vi "GetPort.vi"(8 "error in (no error)":errorcluster, 10 "Port":u8, 11 "NXP LPCXpresso54608 in":refnum<class "NXP LPCXpresso54608.lvclass">) -> (0 "error out":errorcluster, 1 "Response":string, 2 "Value":u8, 3 "NXP LPCXpresso54608 out":refnum<class "NXP LPCXpresso54608.lvclass">)   [LabVIEW 2020, in "NXP LPCXpresso54608.lvclass"]
doc: "Get the status of a digital port on the target device."
uses:
  NXP LPCXpresso54608.lvclass
  MCU/MCU.lvclass
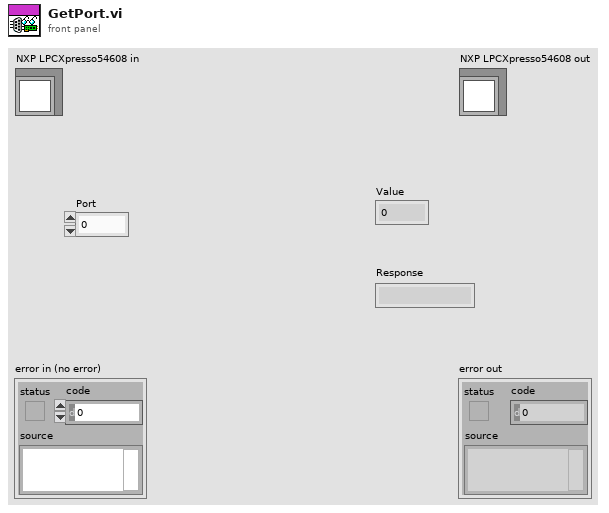
[diagram p1: front panel]
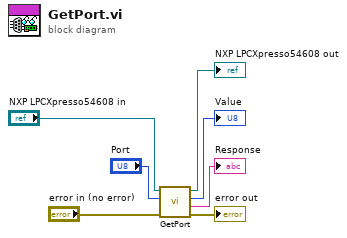
[diagram p0: block diagram]
diagram:
  n1 = call-parent "GetPort.vi"("error in (no error)"="error in (no error)", "Port"="Port", "MCU in"="NXP LPCXpresso54608 in") -> ("error out"=→"error out":errorcluster, "Response"=→"Response":string, "Value"=→"Value":u8, "MCU out"=→"NXP LPCXpresso54608 out":refnum<class "NXP LPCXpresso54608.lvclass">)  [unwired: 5 in]
